vi "PrepareDBPath.vi"(11 "DBLocation":path) -> (3 "result string":string)   [LabVIEW 2020, in "ORM_DBC_Kdb.lvlib" / "DBC.lvclass"]
uses:
  DBC.lvclass
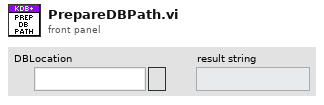
[diagram p1: front panel]
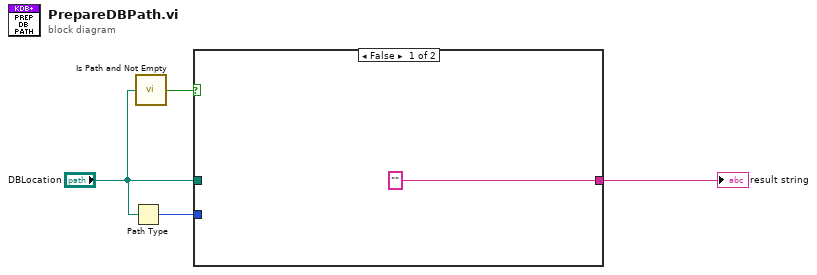
[diagram p0: block diagram]
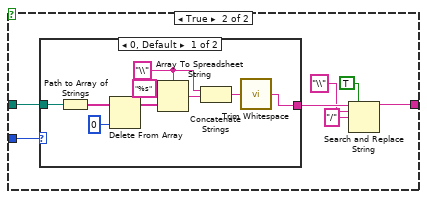
[diagram p2: hidden frame]
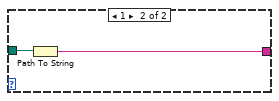
[diagram p3: hidden frame]
diagram:
  n1 = Path Type(1:"DBLocation") -> (0:w4:i16)
  n2 = call <vilib>:"Is Path and Not Empty.vi"("path"="DBLocation") -> ("Is Path and Not Empty?"=w2:bool)  [unwired: 4 in]
  n3 = case shown="False" w2 {
    tunnel: w4 -> [_ w9]
    tunnel: "DBLocation" -> [_ w7]
    tunnel: ["" ("result string") w6] -> w1
    frame False {
    }
    frame True {
      n4 = case shown="0, Default" w9 {
        tunnel: w7 -> [w21 w23]
        tunnel: [w14 w22] -> w10
        frame 0, Default {
          w16 = "\\" ("delimiter (Tab)")
          n5 = Path to Array of Strings(0:w21) -> (2:w20:string[])  [unwired: 1 out]
          n6 = Delete From Array(array=w20, index=0) -> (array with subset deleted=w18:string[])  [unwired: 1 in, 1 out]
          n7 = Array To Spreadsheet String(delimiter (Tab)=w16, array=w18, 3:"%s" ("format string")) -> (spreadsheet string=w17:string)
          n8 = Concatenate Strings(w16, w17) -> (w15:string)
          n9 = call <vilib>:"Trim Whitespace.vi"("string"=w15) -> ("trimmed string"=w14:string)  [unwired: 1 in]
        }
        frame 1 {
          n10 = Path To String(path=w23) -> (string=w22:string)
        }
      }
      n11 = Search and Replace String(replace all?=TRUE ("replace all? (F)"), input string=w10, search string="\\", replace string="/" ("replace string (\"\")")) -> (result string=w6:string)  [unwired: 4 in, 3 out]
    }
  }
  "result string" <- w1
